vi "IR-Correction-Pro_Api.vi"(4 "ExitRange":dbl=0.08, 6 "精準度":dbl=20.0, 7 "目標電壓":dbl[](array[numeric])=[2.00487, 1.87997, 1.94422, 1.88569, 1.82844, 1.91098, 1.88335, 2.08625], 8 "Error In":errorcluster, 9 "副邊校正":T1(ring)=enum."無", 11 "主編校正":enum16{"前", "後", "オ", "右", "無"}(ring)=enum."無") -> (0 "Error Out":errorcluster)   [LabVIEW 2019]
uses:
  <vilib>/Platform/TimedLoop/XDataNode/timing_clust.ctl
  <vilib>/Platform/TimedLoop/XDataNode/nitl_modes.ctl
  <vilib>/Platform/TimedLoop/XDataNode/wakeup.ctl
  <vilib>/Platform/TimedLoop/XDataNode/XDataNode.xnode
  <vilib>/addons/control/pid/pid.llb/PID (DBL Array).vi
  <vilib>/addons/control/pid/NI_PID_pid.lvlib
  <vilib>/Platform/TimedLoop/XDataNode/XDNodeRunTimeDep.lvlib
panel:
  in  "Stop":bool
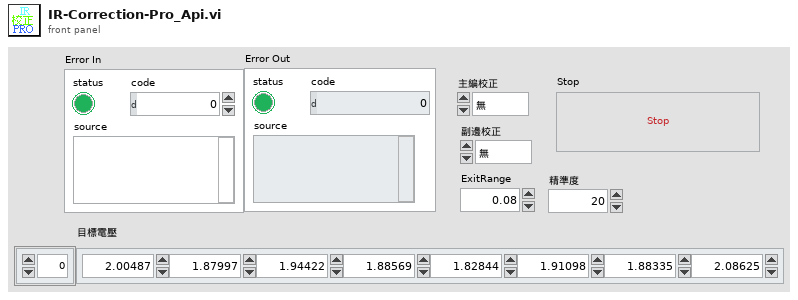
[diagram p1: front panel]
types:
  T1 = enum16{"前", "後", "オ", "右", "無", "0", "1", "2", "3", "4", "5", "6", "7"}
  T2 = cluster{"proportional gain (Kc)":dbl, "integral time (Ti, min)":dbl, "derivative time (Td, min)":dbl}[]
  T3 = typedef "XDNodeRunTimeDep.lvlib/timing_clust.ctl" = cluster{"Expected End [f-1]":u64, "Actual End [f-1]":u64, "Finished Late? [f-1]":bool, "Expected End [i-1]":u64, "Actual End [i-1]":u64, "Finished Late? [i-1]":bool, "Expected Start [i]":u64, "Actual Start [i]":u64, "Expected Start [f]":u64, "Actual Start [f]":u64, "Source Name":string, "Structure Name":string, "Period":i64, "Deadline":i64, "Offset":i64, "Start":i64, "Priority":i32, "Timeout":i32, "Mode":T4, "Wakeup Reason":T5, "Error":errorcluster, "Source Type":string, "Secondary Source Type":string, "Global End Time":u64, "Global Start Time":u64, "Frame Duration":u64, "Iteration Duration":u64, "Assigned CPU":i32, "I/O Scan Engine Mode":u32}
  T4 = typedef "XDNodeRunTimeDep.lvlib/nitl_modes.ctl" = enum32{"No Change", "Process missed periods, maintain original phase", "Discard missed periods, maintain original phase", "Process missed periods, ignore original phase", "Discard missed periods, ignore original phase"}
  T5 = typedef "XDNodeRunTimeDep.lvlib/wakeup.ctl" = enum32{"Normal", "Aborted", "Asynchronous wakeup", "Timing source error", "Timed loop error", "Timeout"}
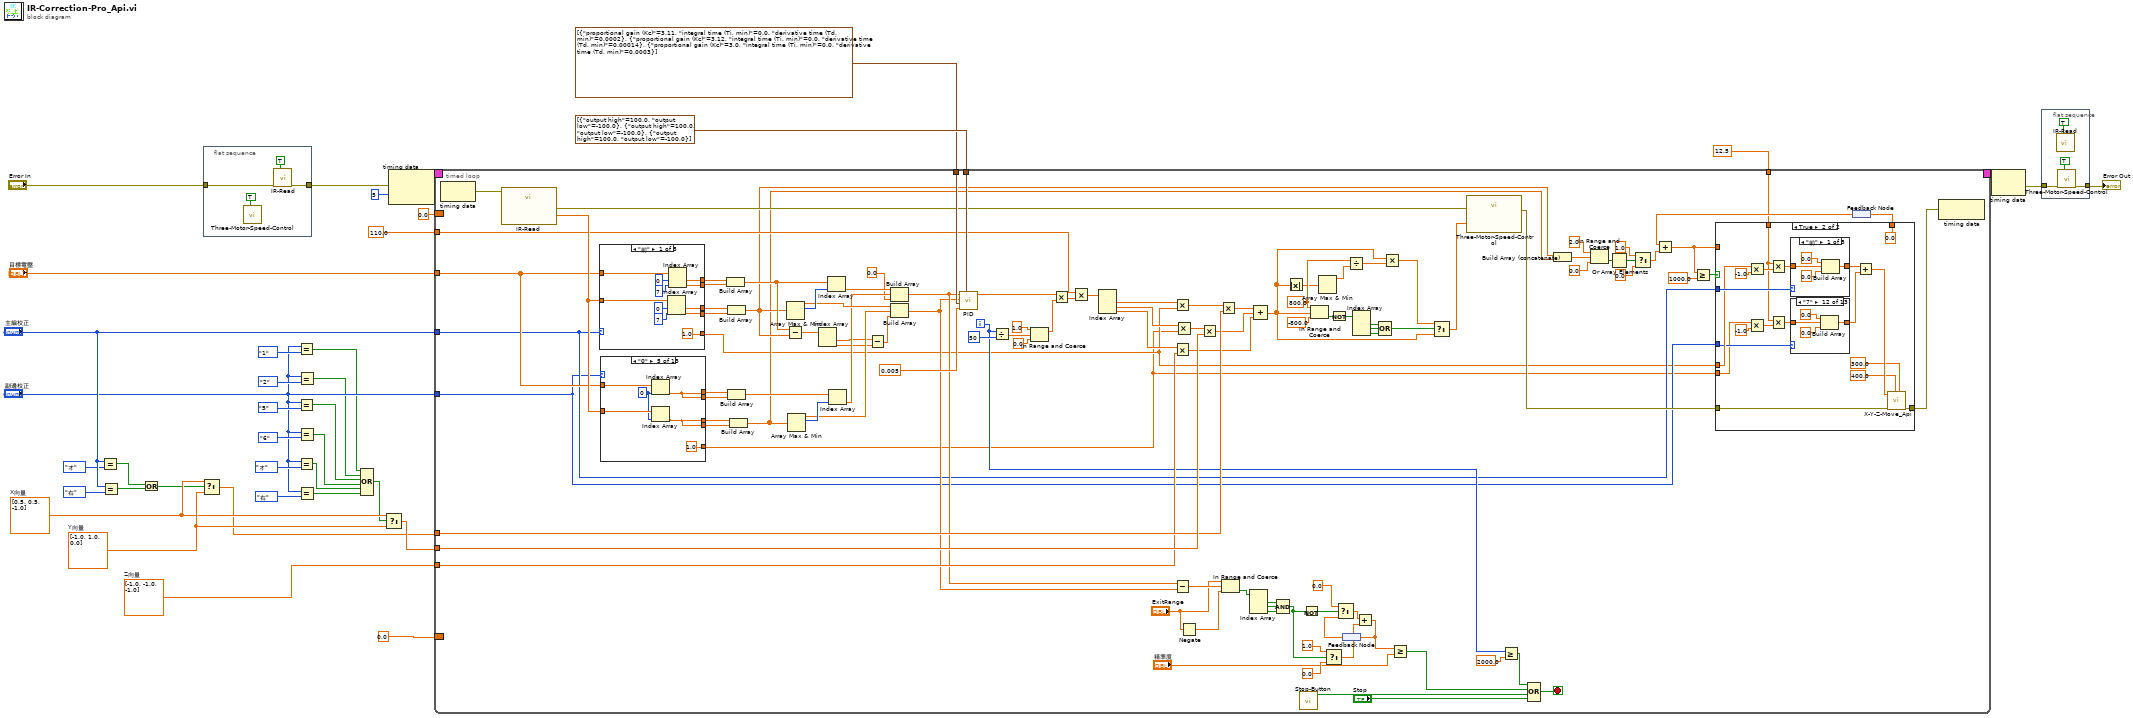
[diagram p0: block diagram]
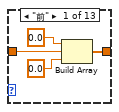
[diagram p3: hidden frame]
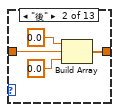
[diagram p4: hidden frame]
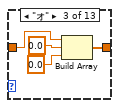
[diagram p5: hidden frame]
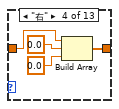
[diagram p6: hidden frame]
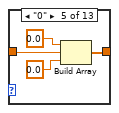
[diagram p7: hidden frame]
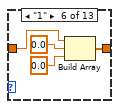
[diagram p8: hidden frame]
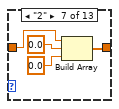
[diagram p9: hidden frame]
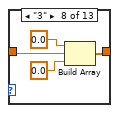
[diagram p10: hidden frame]
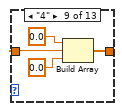
[diagram p11: hidden frame]
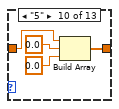
[diagram p12: hidden frame]
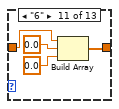
[diagram p13: hidden frame]
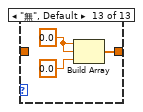
[diagram p14: hidden frame]
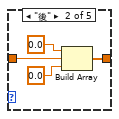
[diagram p15: hidden frame]
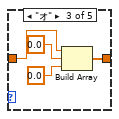
[diagram p16: hidden frame]
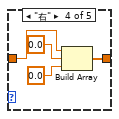
[diagram p17: hidden frame]
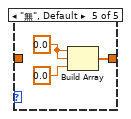
[diagram p18: hidden frame]
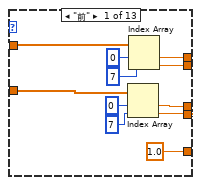
[diagram p19: hidden frame]
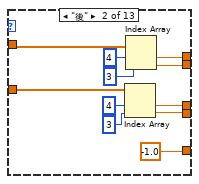
[diagram p20: hidden frame]
diagram:
  w33 = dbl[] [-1.0, -1.0, -1.0]  # Z向量
  w28 = dbl[] [-1.0, 1.0, 0.0]  # Y向量
  w27 = dbl[] [0.5, 0.5, -1.0]  # X向量
  n1 = Equal?(x="主編校正", y=enum16{"前", "後", "オ", "右", "無"}."オ") -> (x = y?=w29:bool)
  n2 = Equal?(x="主編校正", y=enum16{"前", "後", "オ", "右", "無"}."右") -> (x = y?=w30:bool)
  n3 = Or(x=w29, y=w30) -> (x .or. y?=w18:bool)
  n4 = Select(t=w27, s=w18, f=w28) -> (s? t:f=w25:dbl[])
  n5 = flat-sequence {
    tunnel: "Error In" -> [w41]
    tunnel: [w40] -> w22
    frame #0 {
      n6 = call "Three-Motor-Speed-Control.vi"("Reset"=TRUE) -> ()  [unwired: 10 in, 1 out]
      n7 = call "IR-Read.vi"("Reset"=TRUE, "Error In"=w41) -> ("Error Out"=w40:errorcluster)  [unwired: 8 in, 1 out]
    }
  }
  n8 = Equal?(x="副邊校正", y=T1."1") -> (x = y?=w3:bool)
  n9 = Equal?(x="副邊校正", y=T1."5") -> (x = y?=w2:bool)
  n10 = Equal?(x="副邊校正", y=T1."オ") -> (x = y?=w6:bool)
  n11 = Equal?(x="副邊校正", y=T1."2") -> (x = y?=w4:bool)
  n12 = Equal?(x="副邊校正", y=T1."6") -> (x = y?=w5:bool)
  n13 = Equal?(x="副邊校正", y=T1."右") -> (x = y?=w7:bool)
  n14 = Compound Arithmetic op=OR(w3, w4, w2, w5, w6, w7) -> (w1:bool)
  n15 = Select(t=w27, s=w1, f=w28) -> (s? t:f=w26:dbl[])
  n16 = node-c288(w22, i64 5 ("Period")) -> (w39:T3)
  n17 = timed-loop {
    timing: w39 -> [_]
    timing-out: [_] -> w38
    tunnel: "主編校正" -> [w55]
    tunnel: "目標電壓" -> [w138]
    tunnel: "副邊校正" -> [w54]
    tunnel: cluster{"output high":dbl, "output low":dbl}[] [{"output high"=100.0, "output low"=-100.0}, {"output high"=100.0, "output low"=-100.0}, {"output high"=100.0, "output low"=-100.0}] ("output range") -> [w128]
    tunnel: T2 [{"proportional gain (Kc)"=3.11, "integral time (Ti, min)"=0.0, "derivative time (Td, min)"=0.0002}, {"proportional gain (Kc)"=3.12, "integral time (Ti, min)"=0.0, "derivative time (Td, min)"=0.00014}, {"proportional gain (Kc)"=3.0, "integral time (Ti, min)"=0.0, "derivative time (Td, min)"=0.0003}] ("PID gains") -> [w127]
    tunnel: w33 -> [w118]
    tunnel: w26 -> [w121]
    tunnel: w25 -> [w120]
    border: 0.0 -> [_]
    tunnel: 110.0 ("Numeric") -> [w77]
    border: 0.0 -> [_]
    tunnel: 12.5 ("x") -> [w53]
    i -> [w73]
    stop <- w72 stop-if-true
    w46 = 800.0
    n18 = node-c288() -> (w114:errorcluster)  [unwired: 1 in]
    n19 = call "IR-Read.vi"("Error In"=w114) -> ("Error Out"=w103:errorcluster, "輸出紅外線值"=w139:dbl[])  [unwired: 9 in]
    n20 = case shown="\"前\"" w55 {
      tunnel: w138 -> [w349 w355 w366 w382 _]
      tunnel: w139 -> [w348 w354 w365 w378 _]
      tunnel: [w347 w356 w371 w376 w387] -> w152
      tunnel: [w346 w357 w370 w377 w387] -> w151
      tunnel: [w345 w358 w369 w379 w387] -> w150
      tunnel: [w344 w359 w368 w380 w387] -> w149
      tunnel: [1.0 ("y") -1.0 ("y") -1.0 ("y") 1.0 ("y") w387] -> w52
      frame "前" {
        n21 = Index Array(array=w348, index #1=0 ("index"), index #2=7 ("index")) -> (element #1=w345:dbl, element #2=w344:dbl)
        n22 = Index Array(array=w349, index #1=0 ("index"), index #2=7 ("index")) -> (element #1=w347:dbl, element #2=w346:dbl)
      }
      frame "後" {
        n23 = Index Array(array=w354, index #1=4 ("index"), index #2=3 ("index")) -> (element #1=w358:dbl, element #2=w359:dbl)
        n24 = Index Array(array=w355, index #1=4 ("index"), index #2=3 ("index")) -> (element #1=w356:dbl, element #2=w357:dbl)
      }
      frame "オ" {
        n25 = Index Array(array=w365, index #1=2 ("index"), index #2=1 ("index")) -> (element #1=w369:dbl, element #2=w368:dbl)
        n26 = Index Array(array=w366, index #1=2 ("index"), index #2=1 ("index")) -> (element #1=w371:dbl, element #2=w370:dbl)
      }
      frame "右" {
        n27 = Index Array(array=w378, index #1=6 ("index"), index #2=5 ("index")) -> (element #1=w379:dbl, element #2=w380:dbl)
        n28 = Index Array(array=w382, index #1=6 ("index"), index #2=5 ("index")) -> (element #1=w376:dbl, element #2=w377:dbl)
      }
      frame "無", Default {
        w387 = 0.0 ("Numeric")
      }
    }
    n29 = case shown="\"0\"" w54 {
      tunnel: w138 -> [w251 w257 w271 w284 w294 w300 w306 w312 w318 w324 w330 w336 _]
      tunnel: w139 -> [w250 w256 w272 w283 w291 w297 w304 w310 w316 w321 w327 w334 _]
      tunnel: [w249 w258 w274 w282 w293 w299 w303 w308 w314 w323 w329 w332 w337] -> w140
      tunnel: [w248 w259 w268 w281 w293 w299 w303 w308 w314 w323 w329 w332 w337] -> w141
      tunnel: [w247 w260 w273 w280 w289 w295 w302 w307 w313 w319 w325 w331 w337] -> w142
      tunnel: [w246 w261 w267 w279 w289 w295 w302 w307 w313 w319 w325 w331 w337] -> w143
      tunnel: [1.0 ("y") -1.0 ("y") -1.0 ("y") 1.0 ("y") 1.0 ("Numeric") -1.0 ("Numeric") -1.0 ("Numeric") -1.0 ("Numeric") -1.0 ("Numeric") 1.0 ("Numeric") 1.0 ("Numeric") 1.0 ("Numeric") w337] -> w51
      frame "前" {
        n30 = Index Array(array=w250, index #1=0 ("index"), index #2=7 ("index")) -> (element #1=w247:dbl, element #2=w246:dbl)
        n31 = Index Array(array=w251, index #1=0 ("index"), index #2=7 ("index")) -> (element #1=w249:dbl, element #2=w248:dbl)
      }
      frame "後" {
        n32 = Index Array(array=w256, index #1=4 ("index"), index #2=3 ("index")) -> (element #1=w260:dbl, element #2=w261:dbl)
        n33 = Index Array(array=w257, index #1=4 ("index"), index #2=3 ("index")) -> (element #1=w258:dbl, element #2=w259:dbl)
      }
      frame "オ" {
        n34 = Index Array(array=w272, index #1=2 ("index"), index #2=1 ("index")) -> (element #1=w273:dbl, element #2=w267:dbl)
        n35 = Index Array(array=w271, index #1=2 ("index"), index #2=1 ("index")) -> (element #1=w274:dbl, element #2=w268:dbl)
      }
      frame "右" {
        n36 = Index Array(array=w283, index #1=6 ("index"), index #2=5 ("index")) -> (element #1=w280:dbl, element #2=w279:dbl)
        n37 = Index Array(array=w284, index #1=6 ("index"), index #2=5 ("index")) -> (element #1=w282:dbl, element #2=w281:dbl)
      }
      frame "0" {
        w290 = 0 ("index")
        n38 = Index Array(array=w294, index=w290) -> (element=w293:dbl)
        n39 = Index Array(array=w291, index=w290) -> (element=w289:dbl)
      }
      frame "1" {
        w296 = 1 ("index")
        n40 = Index Array(array=w300, index=w296) -> (element=w299:dbl)
        n41 = Index Array(array=w297, index=w296) -> (element=w295:dbl)
      }
      frame "2" {
        w301 = 2 ("index")
        n42 = Index Array(array=w306, index=w301) -> (element=w303:dbl)
        n43 = Index Array(array=w304, index=w301) -> (element=w302:dbl)
      }
      frame "3" {
        w309 = 3 ("index")
        n44 = Index Array(array=w312, index=w309) -> (element=w308:dbl)
        n45 = Index Array(array=w310, index=w309) -> (element=w307:dbl)
      }
      frame "4" {
        w315 = 4 ("index")
        n46 = Index Array(array=w318, index=w315) -> (element=w314:dbl)
        n47 = Index Array(array=w316, index=w315) -> (element=w313:dbl)
      }
      frame "5" {
        w320 = 5 ("index")
        n48 = Index Array(array=w324, index=w320) -> (element=w323:dbl)
        n49 = Index Array(array=w321, index=w320) -> (element=w319:dbl)
      }
      frame "6" {
        w326 = 6 ("index")
        n50 = Index Array(array=w330, index=w326) -> (element=w329:dbl)
        n51 = Index Array(array=w327, index=w326) -> (element=w325:dbl)
      }
      frame "7" {
        w333 = 7 ("index")
        n52 = Index Array(array=w336, index=w333) -> (element=w332:dbl)
        n53 = Index Array(array=w334, index=w333) -> (element=w331:dbl)
      }
      frame "無", Default {
        w337 = 0.0 ("Numeric")
      }
    }
    n54 = Build Array(w152, w151) -> (w133:dbl[])
    n55 = Build Array(w150, w149) -> (w71:dbl[])
    n56 = Build Array(w140, w141) -> (w144:dbl[])
    n57 = Build Array(w142, w143) -> (w70:dbl[])
    n58 = Array Max & Min(array=w71) -> (max value=w146:dbl, max index (indices)=w148:i32)  [unwired: 2 out]
    n59 = Subtract(x=w133, y=w71) -> (x-y=w132:dbl[])
    n60 = Array Max & Min(array=w70) -> (max value=w135:dbl, max index (indices)=w145:i32)  [unwired: 2 out]
    n61 = Index Array(array=w132) -> (element #1=w131:dbl, element #2=w130:dbl)  [unwired: 2 in]
    n62 = Index Array(array=w133, index=w148) -> (element=w147:dbl)
    n63 = Index Array(array=w144, index=w145) -> (element=w136:dbl)
    n64 = Subtract(x=w131, y=w130) -> (x-y=w129:dbl)
    n65 = Build Array(w147, w136, 0.0 ("element")) -> (w101:dbl[])
    n66 = Build Array(w146, w135, w129) -> (w100:dbl[])
    n67 = call-poly <vilib>:"PID.vi"("output range"=w128, "dt (s)"=0.005, "PID gains"=w127, "process variable"=w100, "setpoint"=w101) -> ("output"=w80:dbl[])  [unwired: 5 in, 1 out]
    n68 = Divide(x=w73, y=50) -> (x/y=w84:dbl)
    n69 = In Range and Coerce(upper limit=1.0, x=w84, lower limit=0.0) -> (coerced(x)=w81:dbl)  [unwired: 1 out]
    n70 = Multiply(x=w80, y=w81) -> (x*y=w78:dbl[])
    n71 = Multiply(x=w77, y=w78) -> (x*y=w79:dbl[])
    n72 = Index Array(array=w79) -> (element #1=w125:dbl, element #2=w124:dbl, element #3=w119:dbl)  [unwired: 3 in]
    n73 = Multiply(x=w125, y=w52) -> (x*y=w123:dbl)
    n74 = Multiply(x=w119, y=w118) -> (x*y=w115:dbl[])
    n75 = Subtract(x=w101, y=w100) -> (x-y=w102:dbl[])
    n76 = Multiply(x=w124, y=w51) -> (x*y=w122:dbl)
    n77 = Negate(x="ExitRange") -> (-x=w48:dbl)
    n78 = Multiply(x=w122, y=w121) -> (x*y=w116:dbl[])
    n79 = Multiply(x=w123, y=w120) -> (x*y=w117:dbl[])
    n80 = In Range and Coerce(upper limit="ExitRange", x=w102, lower limit=w48) -> (In Range?=w99:bool[])  [unwired: 1 out]
    n81 = Index Array(array=w99) -> (element #1=w98:bool, element #2=w97:bool, element #3=w96:bool)  [unwired: 3 in]
    n82 = Compound Arithmetic op=ADD(w117, w116, w115) -> (w44:dbl[])
    n83 = Compound Arithmetic op=AND(w98, w97, w96) -> (w90:bool)
    n84 = Absolute Value(x=w44) -> (abs(x)=w45:dbl[])
    n85 = call "Stop-Button.vi"() -> ("顯示按下?"=w137:bool)  [unwired: 10 in, 1 out]
    n86 = Not(x=w90) -> (.not. x?=w91:bool)
    n87 = In Range and Coerce(upper limit=w46, x=w44, lower limit=-800.0) -> (In Range?=w112:bool[])  [unwired: 1 out]
    n88 = Array Max & Min(array=w45) -> (max value=w76:dbl)  [unwired: 3 out]
    n89 = Select(t=1.0, s=w90, f=0.0) -> (s? t:f=w93:dbl)
    n90 = Not(x=w112) -> (.not. x?=w111:bool[])
    n91 = feedback #1() -> (w92:dbl)
    n92 = Select(t=0.0, s=w91, f=w92) -> (s? t:f=w88:dbl)
    n93 = Divide(x=w46, y=w76) -> (x/y=w105:dbl)
    n94 = Index Array(array=w111) -> (element #1=w110:bool, element #2=w109:bool, element #3=w108:bool)  [unwired: 3 in]
    n95 = Add(x=w88, y=w93) -> (x+y=w87:dbl)
    n96 = feedback-in #1(w87) -> ()
    n97 = Compound Arithmetic op=OR(w110, w109, w108) -> (w107:bool)
    n98 = Multiply(x=w44, y=w105) -> (x*y=w104:dbl[])
    n99 = Greater Or Equal?(x=w87, y="精準度") -> (x >= y?=w86:bool)
    n100 = Select(t=w104, s=w107, f=w44) -> (s? t:f=w106:dbl[])
    n101 = call "Three-Motor-Speed-Control.vi"("Error In"=w103, "速度(秒/度)"=w106) -> ("Error Out"=w57:errorcluster)  [unwired: 9 in]
    n102 = Greater Or Equal?(x=w73, y=2000.0) -> (x >= y?=w75:bool)
    n103 = Compound Arithmetic op=OR(w75, w86, w137, "Stop") -> (w72:bool)
    n104 = Build Array (concatenate)(w71, w70) -> (w69:dbl[])
    n105 = In Range and Coerce(upper limit=2.0 ("dt (s)"), x=w69, lower limit=0.0 ("dt (s)")) -> (In Range?=w66:bool[])  [unwired: 1 out]
    n106 = Or Array Elements(Boolean array=w66) -> (logical OR=w65:bool)
    n107 = Select(t=1.0, s=w65, f=0.0 ("t")) -> (s? t:f=w62:dbl)
    n108 = feedback #2() -> (w60:dbl)
    n109 = Add(x=w60, y=w62) -> (x+y=w59:dbl)
    n110 = Greater Or Equal?(x=w59, y=1000.0) -> (x >= y?=w50:bool)
    n111 = case shown="True" w50 {
      tunnel: [w155 0.0] -> w61
      tunnel: w59 -> [w155 _]
      tunnel: w57 -> [w154 w173]
      tunnel: [w154 w172] -> w56
      tunnel: w55 -> [_ w171]
      tunnel: w54 -> [_ w163]
      tunnel: w53 -> [_ w161]
      tunnel: w52 -> [_ w169]
      tunnel: w51 -> [_ w162]
      frame False {
      }
      frame True {
        n112 = Multiply(x=w169, y=-1.0) -> (x*y=w170:dbl)
        n113 = Multiply(x=w162, y=-1.0) -> (x*y=w164:dbl)
        n114 = Multiply(x=w161, y=w170) -> (x*y=w167:dbl)
        n115 = Multiply(x=w161, y=w164) -> (x*y=w166:dbl)
        n116 = case shown="\"前\"" w171 {
          tunnel: w167 -> [w229 w233 w235 w239 _]
          tunnel: [w226 w230 w234 w238 w242] -> w160
          frame "前" {
            n117 = Build Array(0.0 ("element"), w229, 0.0 ("element")) -> (w226:dbl[])
          }
          frame "後" {
            n118 = Build Array(0.0 ("element"), w233, 0.0 ("element")) -> (w230:dbl[])
          }
          frame "オ" {
            n119 = Build Array(w235, 0.0 ("element"), 0.0 ("element")) -> (w234:dbl[])
          }
          frame "右" {
            n120 = Build Array(w239, 0.0 ("element"), 0.0 ("element")) -> (w238:dbl[])
          }
          frame "無", Default {
            w243 = 0.0 ("element")
            n121 = Build Array(w243, w243, 0.0 ("element")) -> (w242:dbl[])
          }
        }
        n122 = case shown="\"7\"" w163 {
          tunnel: w166 -> [w178 w182 w183 w187 w192 w196 w199 w204 w208 w211 w215 w219 _]
          tunnel: [w175 w179 w184 w188 w191 w195 w200 w203 w207 w212 w216 w220 w223] -> w159
          frame "前" {
            n123 = Build Array(0.0 ("element"), w178, 0.0 ("element")) -> (w175:dbl[])
          }
          frame "後" {
            n124 = Build Array(0.0 ("element"), w182, 0.0 ("element")) -> (w179:dbl[])
          }
          frame "オ" {
            n125 = Build Array(w183, 0.0 ("element"), 0.0 ("element")) -> (w184:dbl[])
          }
          frame "右" {
            n126 = Build Array(w187, 0.0 ("element"), 0.0 ("element")) -> (w188:dbl[])
          }
          frame "0" {
            n127 = Build Array(0.0 ("element"), w192, 0.0 ("element")) -> (w191:dbl[])
          }
          frame "1" {
            n128 = Build Array(w196, 0.0 ("element"), 0.0 ("element")) -> (w195:dbl[])
          }
          frame "2" {
            n129 = Build Array(w199, 0.0 ("element"), 0.0 ("element")) -> (w200:dbl[])
          }
          frame "3" {
            n130 = Build Array(0.0 ("element"), w204, 0.0 ("element")) -> (w203:dbl[])
          }
          frame "4" {
            n131 = Build Array(0.0 ("element"), w208, 0.0 ("element")) -> (w207:dbl[])
          }
          frame "5" {
            n132 = Build Array(w211, 0.0 ("element"), 0.0 ("element")) -> (w212:dbl[])
          }
          frame "6" {
            n133 = Build Array(w215, 0.0 ("element"), 0.0 ("element")) -> (w216:dbl[])
          }
          frame "7" {
            n134 = Build Array(0.0 ("element"), w219, 0.0 ("element")) -> (w220:dbl[])
          }
          frame "無", Default {
            w224 = 0.0 ("element")
            n135 = Build Array(w224, w224, 0.0 ("element")) -> (w223:dbl[])
          }
        }
        n136 = Add(x=w160, y=w159) -> (x+y=w158:dbl[])
        n137 = call "X-Y-Z-Move_Api.vi"("加速度"=300.0, "最高速"=400.0, "Error In"=w173, "X-Y-Z移動"=w158) -> ("Error Out"=w172:errorcluster)  [unwired: 6 in, 1 out]
      }
    }
    n138 = feedback-in #2(w61) -> ()
    n139 = node-c288(w56) -> ()  [unwired: 1 out]
  }
  n140 = node-c288(w38) -> (w21:errorcluster)
  n141 = flat-sequence {
    tunnel: [w391] -> w20
    tunnel: w21 -> [w388]
    frame #0 {
      n142 = call "IR-Read.vi"("Reset"=TRUE) -> ()  [unwired: 9 in, 2 out]
      n143 = call "Three-Motor-Speed-Control.vi"("Reset"=TRUE, "Error In"=w388) -> ("Error Out"=w391:errorcluster)  [unwired: 9 in]
    }
  }
  "Error Out" <- w20
